vi "Are Analog Waveforms Equal.vi"(1 "waveform 2":waveform(dbl)={"t0"=timestamp(0 s since 1904-01-01), "dt"=0.0, "Y"=[]}, 2 "waveform":waveform(dbl)={"t0"=timestamp(0 s since 1904-01-01), "dt"=0.0, "Y"=[]}) -> (0 "waveforms equal":bool)   [LabVIEW 2013]
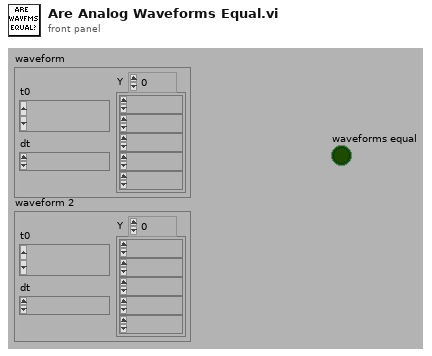
[diagram p1: front panel]
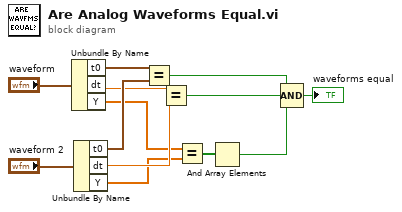
[diagram p0: block diagram]
diagram:
  n1 = Unbundle By Name("waveform") -> ("t0"=w11:timestamp, "dt"=w9:dbl, "Y"=w7:dbl[])
  n2 = Unbundle By Name("waveform 2") -> ("t0"=w10:timestamp, "dt"=w8:dbl, "Y"=w6:dbl[])
  n3 = Equal?(x=w11, y=w10) -> (x = y?=w4:bool)
  n4 = Equal?(x=w9, y=w8) -> (x = y?=w3:bool)
  n5 = Equal?(x=w7, y=w6) -> (x = y?=w5:bool[])
  n6 = And Array Elements(Boolean array=w5) -> (logical AND=w2:bool)
  n7 = Compound Arithmetic op=AND(w4, w3, w2) -> (→"waveforms equal":bool)
